vi "test_vision.vi"() -> ()   [LabVIEW 2021]
uses:
  <vilib>/myRIO/Common/Instrument Driver Framework/myRIO v1.0/UART/vis/myRIO v1.0 Close UART.vi
  <vilib>/myRIO/Common/Instrument Driver Framework/Utilities/vis/FPGA Ref Manager.vi
  <vilib>/myRIO/Common/Instrument Driver Framework/myRIO v1.0/myRIO v1.0 Reset FPGA.vi
  <vilib>/myRIO/Common/Instrument Driver Framework/myRIO v1.0/IRQ/vis/myRIO v1.0 IRQ Info FGV.vi
  <vilib>/myRIO/Common/Instrument Driver Framework/myRIO v1.0/IRQ/vis/myRIO v1.0 Timer IRQ Info FGV.vi
  <vilib>/myRIO/Common/Instrument Driver Framework/myRIO v1.0/IRQ/vis/myRIO v1.0 ISR Agent.vi
  <vilib>/myRIO/Instrument Drivers/Utilities/vis/Reset Index.vi
  <vilib>/myRIO/Common/Instrument Driver Framework/myRIO v1.0/Resource Manager/vis/myRIO v1.0 Block Write Resource Manager.vi
  <vilib>/myRIO/Instrument Drivers/Utilities/Utilities.lvlib
panel:
  out "error out":errorcluster
  out "Ball_Coordinates":dbl[](array[numeric])
  in  "stop":bool
  out "Tick Count(uSec)":u32
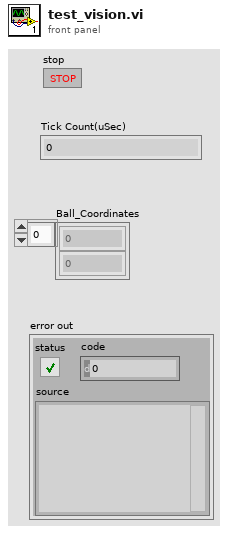
[diagram p1: front panel]
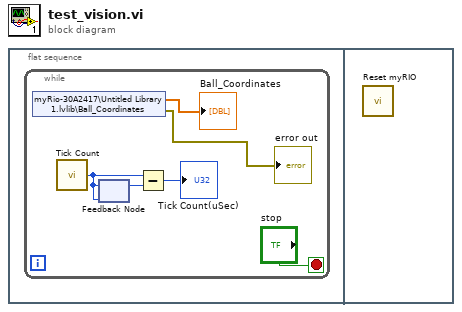
[diagram p0: block diagram]
diagram:
  n1 = flat-sequence {
    frame #0 {
      n2 = while {
        stop <- "stop" stop-if-true
        n3 = shared-variable "myRio-30A2417\\Untitled Library 1.lvlib\\Ball_Coordinates"() -> (→"Ball_Coordinates":dbl[], error out=→"error out":errorcluster)  [unwired: 1 in]
        n4 = call "Tick Count"() -> ("Tick Count(uSec)"=w5:u32)
        n5 = feedback-in #1(w5) -> ()
        n6 = feedback #1(w5) -> (w4:u32)
        n7 = Subtract(x=w5, y=w4) -> (x-y=→"Tick Count(uSec)":u32)
      }
    }
    frame #1 {
      n8 = call <vilib>:"Reset myRIO.vi"() -> ()  [unwired: 11 in, 1 out]
    }
  }
